vi "Transform.vi"(7 "Type X":T1(ring), 8 "error in (no error)":errorcluster caption="entrée d'erreur (pas d'erreur)", 9 "y":string[][](array[string]), 10 "X":string[][](array[string]), 11 "Normalizer.lvclass":refnum<class "Normalizer.lvclass">) -> (0 "error out":errorcluster caption="sortie d'erreur", 2 "Data":T2, 3 "Normalizer.lvclass":refnum<class "Normalizer.lvclass">)   [LabVIEW 2020, in "Normalizer.lvclass"]
doc: "Scale each non zero row of X to unit norm\n\nReturns : \n\n- X_new : ndarray array of shape (n_samples, n_features_new)\nTransformed array."
uses:
  Normalizer.lvclass
  Normalizer.lvclass/Normalizer.ctl
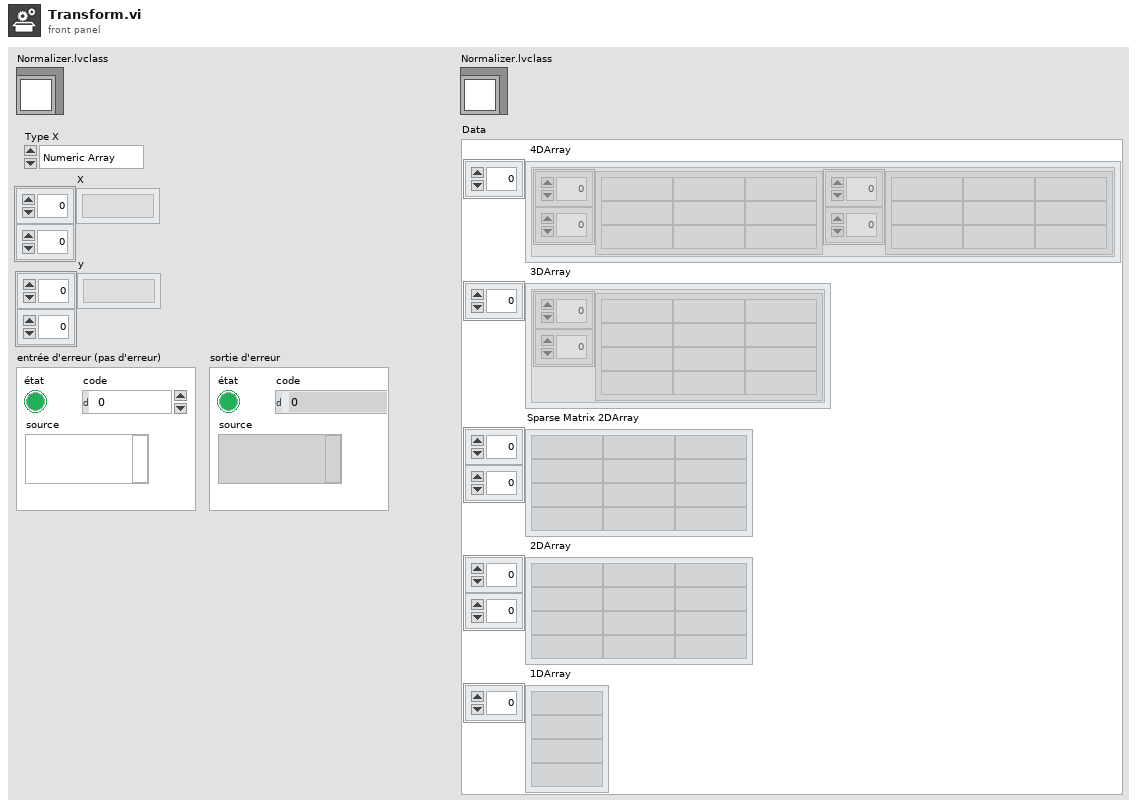
[diagram p1: front panel]
types:
  T1 = enum16{"Numeric Array", "String Array", "Sparse"}
  T2 = cluster{" 4DArray":cluster{"1":string[][], "2":string[][]}[], " 3DArray":cluster{"Tableau":string[][]}[], "Sparse Matrix 2DArray":string[][], " 2DArray":string[][], " 1DArray":string[]}
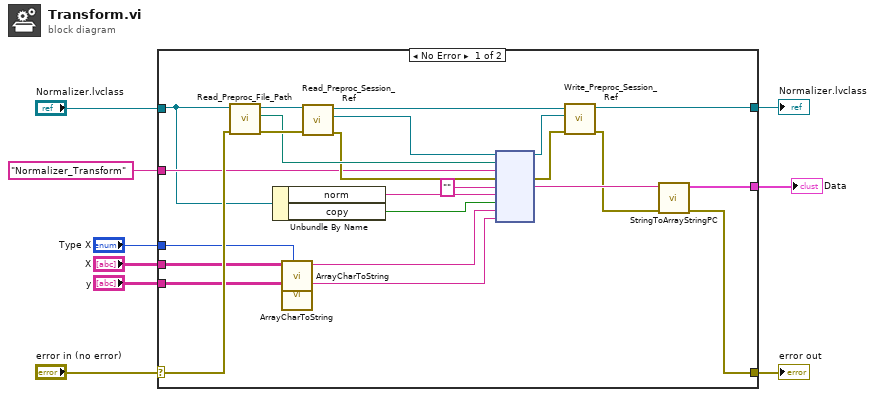
[diagram p0: block diagram]
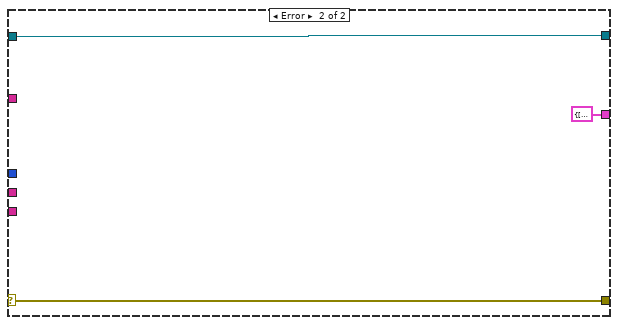
[diagram p2: hidden frame]
diagram:
  n1 = case shown="No Error" "error in (no error)" {
    selector: "error in (no error)" -> [w22 w36]
    tunnel: [w12 w36] -> w8
    tunnel: [w11 w35] -> w6
    tunnel: "Normalizer.lvclass" -> [w20 w35]
    tunnel: "Normalizer_Transform" ("Fonction") -> [w21 _]
    tunnel: [w10 T2 {" 4DArray"=[], " 3DArray"=[], "Sparse Matrix 2DArray"=[], " 2DArray"=[], " 1DArray"=[]} ("Data")] -> w1
    tunnel: "X" -> [w18 _]
    tunnel: "y" -> [w17 _]
    tunnel: "Type X" -> [w19 _]
    frame No Error {
      n2 = call-dynamic "Read_Preproc_File_Path.vi"("error in (no error)"=w22, "Python in"=w20) -> ("error out"=w32:errorcluster, "File_Path"=w29:path, "Python out"=w33:refnum<class "Normalizer.lvclass">)  [unwired: 7 in]
      n3 = Unbundle By Name(w20) -> ("norm"=w24:string, "copy"=w23:bool)
      n4 = call "ArrayCharToString.vi"("Type"=w19, "TAB"=w18) -> ("Instruction"=w16:string)  [unwired: 9 in]
      n5 = call "ArrayCharToString.vi"("TAB"=w17) -> ("Instruction"=w15:string)  [unwired: 10 in]
      n6 = call-dynamic "Read_Preproc_Session_Ref.vi"("error in (no error)"=w32, "Python in"=w33) -> ("error out"=w28:errorcluster, "Session_ref"=w30:refnum<k35>, "Python out"=w31:refnum<class "Normalizer.lvclass">)  [unwired: 7 in]
      n7 = node(w30, w29, w21, w28, "", w24, w23, w16, w15) -> (w26:refnum<k35>, w27:errorcluster, w14:string)  [unwired: 4 in, 2 out]
      n8 = call-dynamic "Write_Preproc_Session_Ref.vi"("error in (no error)"=w27, "Session_ref"=w26, "Python in"=w31) -> ("error out"=w13:errorcluster, "Python out"=w11:refnum<class "Normalizer.lvclass">)  [unwired: 7 in]
      n9 = call "StringToArrayStringPC.vi"("sortie d'erreur"=w13, "Return value"=w14) -> ("sortie d'erreur"=w12:errorcluster, "Data"=w10:T2)  [unwired: 8 in]
    }
    frame Error {
    }
  }
  "error out" <- w8
  "Normalizer.lvclass" <- w6
  "Data" <- w1
